vi "Dashboard Main.vi"() -> ()   [LabVIEW 2015]
uses:
  <vilib>/Utility/miscctls.llb/LVRowAndColumnTypeDef.ctl
  <vilib>/event_ctls.llb/eventvkey.ctl
  <vilib>/Rock Robotics/WPI/Dashboard/WPI_DashboardLogging Global.vi
  <vilib>/Rock Robotics/Network Tables/NT Read Numeric Array.vi
  <vilib>/Rock Robotics/Network Tables/SD Write Number.vi
  <vilib>/Rock Robotics/Network Tables/SD Write Boolean.vi
  <vilib>/Rock Robotics/Network Tables/NT Write Boolean.vi
  <vilib>/Utility/config.llb/Write Key (String).vi
  <vilib>/Utility/config.llb/Write Key (I32).vi
  <vilib>/Utility/config.llb/NI_LVConfig.lvlib
panel:
  in  "Vision 2":u16(ring)=3 items=["IP Camera"=3]
  out "Camera Image 2":T1(plugin-control)
  in  "TCP":refnum<k5>
  in  "Rec Mode":enum32{"Stop", "Record", "Playback"}(radio)
  in  "Vision":u16(ring)=1 items=["USB Cam"=1]
  out "Camera IP":string
  out "Image Message":string="Timeout in Camera Communications"
  in  "Dashboard Tab":T2(tab)
  out "X-Accelerometer":dbl
  in  "Select Auto":string(combo)
  out "NT Connection":bool
  in  "Camera Settings":T3={"Frame Rate"=30, "Compression"=30, "Size"=1} {"Frame Rate" scale=1.0..30.0; "Size" items=["640x480", "320x240", "160x120"]}
  out "MotorChart R":cluster{"Numeric":dbl, "Numeric":dbl}(graph)
  out "MotorChart L":T4(graph)
  out "MotorSliders R":cluster{"MotorSlide1":dbl, "MotorSlide2":dbl} {"MotorSlide2" scale=-1.0..1.0 scale format="%#_2e"; "MotorSlide1" scale=-1.0..1.0 scale format="%#_2e"}
  out "MotorSliders L":T5 {"MotorSlide4 2" scale=0.0..14.0 scale format="%#_2e"; "MotorSlide2" scale=-1.0..1.0 scale format="%#_2e"; "MotorSlide1" scale=-1.0..1.0 scale format="%#_2e"}
  out "JS1 Z":dbl(slide) scale=-1.0..1.0 scale format="%#_2e"
  out "JS1 Graph":cluster{"X":dbl, "Y":dbl}[](graph)
  out "JS1 Buttons":T6
  out "JS2 Z":dbl(slide) scale=-1.0..1.0 scale format="%#_2e"
  out "JS2 Graph":cluster{"X":dbl, "Y":dbl}[](graph)
  out "JS2 Buttons":T6
  out "Mode":T7(ring)=enum."Auto Disabled"
  in  "DB Camera Config":bool
  out "fps":dbl format="%#.1g"
  out "Mbps":dbl format="%#.1g"
  out "Mbps LED":bool
  out "Camera IP 2":string
  in  "Autonomous Select":T8(ring)
  in  "Speed Control":bool
  in  "Top Speed":dbl min=-1.0 max=1.0 step=0.01
  in  "Back Speed":dbl min=-1.0 max=1.0 step=0.01
  out "Gyro":dbl(knob) scale=0.0..360.0
  in  "Intake Speed":dbl min=-1.0 max=1.0 step=0.01
  in  "Gyro Reset":bool
  out "Z-Accelerometer":dbl
  out "Y-Accelerometer":dbl
  in  "DB/String 9":string
  in  "DB/String 8":string
  in  "DB/String 7":string
  in  "DB/String 6":string
  in  "DB/String 5":string
  in  "DB/String 4":string
  in  "DB/String 3":string
  in  "DB/String 2":string
  in  "DB/String 1":string
  in  "DB/String 0":string
  in  "DB/Slider 0":dbl(slide) scale=0.0..5.0
  in  "DB/Slider 1":dbl(slide) scale=0.0..5.0
  in  "DB/Slider 2":dbl(slide) scale=0.0..5.0
  in  "DB/Slider 3":dbl(slide) scale=0.0..5.0
  out "DB/LED 3":bool
  out "DB/LED 2":bool
  out "DB/LED 1":bool
  out "DB/LED 0":bool
  in  "DB/Button 3":bool
  in  "DB/Button 2":bool
  in  "DB/Button 1":bool
  in  "DB/Button 0":bool caption="New Name"
  out "Mbps 2":dbl format="%#.1g"
  in  "Camera Settings 2":T3={"Frame Rate"=30, "Compression"=30, "Size"=1} {"Frame Rate" scale=1.0..30.0; "Size" items=["640x480", "320x240", "160x120"]}
  out "fps 2":dbl format="%#.1g"
  in  "Rec Mode 2":enum32{"Stop", "Record", "Playback"}(radio)
  in  "Test Slider":dbl(slide) scale=0.0..100.0 scale format="%#_3g"
  in  "On/Off":bool caption="Solenoid"
  in  "Test Name":u16(ring) items=["Select the test to run..."]
  in  "Test Tree":string(tree)
  in  "Motor":cluster{"Value":dbl, "Enable":bool} {"Value" scale=-1.0..1.0 scale format="%#_3g"}
  out "Progress":T9 {"Test Progress" scale=0.0..100.0}
  in  "Rev/Fwd":cluster{"Forward":bool, "Reverse":bool}
  in  "Test Ring":u16(ring) items=["Monochrome", "Color"]
  out "Cmd Status":string
  in  "Execute Command":bool
  in  "Command Params":string[][](table)
  in  "Command Selection":i32(listbox)
  in  "CheckList":i32(listbox)
  out "Tree":string(tree)
  out "Camera Image":T1(plugin-control)
  out "Background":bool
  # "Left"
  # "Front"
  # "Right"
  # "Battery"
  # "This tab is a great place for autonomous settings and robot-specific values.\nPlace controls and indicators inside this tab and match name to\nDashboard Variables on robot. You can also delete this comment."
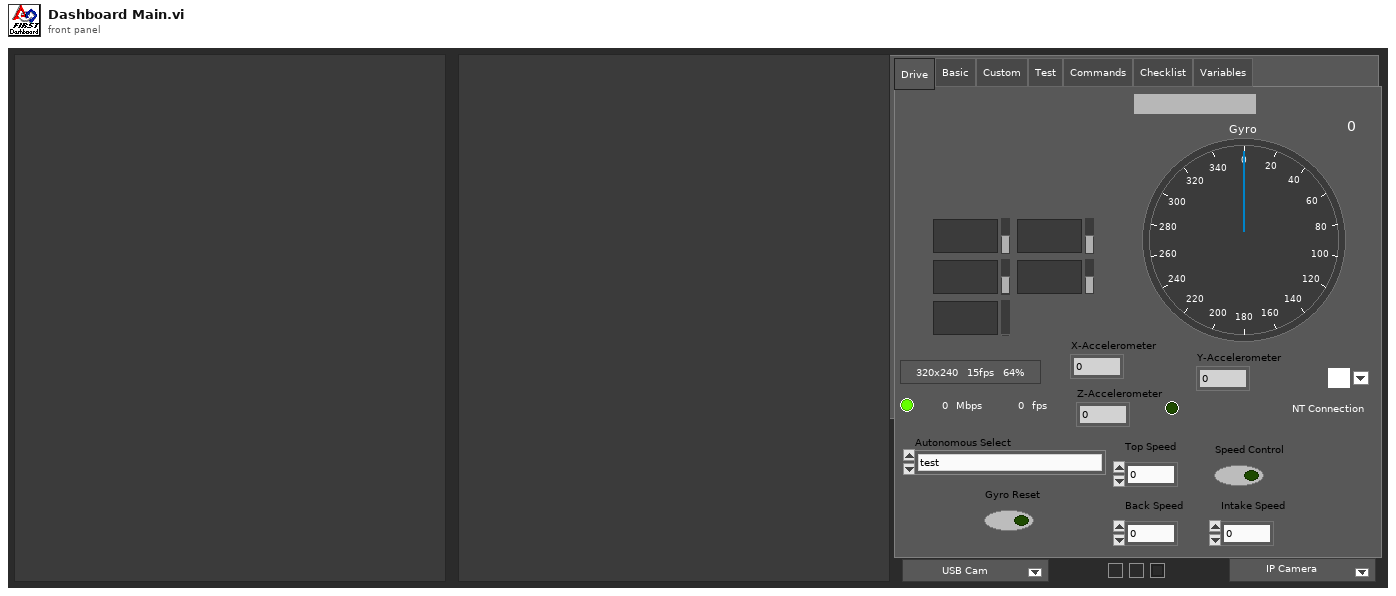
[diagram p1: front panel]
types:
  T1 = typedef "IMAQ Image.ctl" = refnum<image>
  T2 = enum32{"Drive", "Basic", "Custom", "Test", "Commands", "Checklist", "Variables"}
  T3 = cluster{"Frame Rate":i32, "Compression":i32, "Size":u16}
  T4 = cluster{"Numeric":dbl, "Numeric":dbl, "Battery V":dbl}
  T5 = cluster{"MotorSlide1":dbl, "MotorSlide2":dbl, "MotorSlide4 2":dbl}
  T6 = cluster{bool, bool, bool, bool, bool, bool, bool, bool, bool, bool, bool, bool}
  T7 = enum8{"Tele-Op Disabled", "Tele-Op Enabled", "Auto Disabled", "Auto Enabled", "Test Disabled", "Test Enabled", "Disconnected", "No Code", "E-Stop"}
  T8 = enum16{"test", "p value auto", "Ball Variable Shooter", "auto 3"}
  T9 = cluster{"Test Progress":u8, "Test Progress Text":string}
  T10 = typedef "Image Type" = u32
  T11 = cluster{"IDs":cluster{"RPC field ID":u16, "Unique ID":u16}, "String":string}
  T12 = enum32{"Drive", "Basic", "Custom", "Test", "Checklist", "Variables"}
  T13 = cluster{"Camera Image":refnum<vi>, "Dashboard Tab":refnum<vi>, "Background":refnum<vi>, "Vision":refnum<vi>, "Rec Mode":refnum<vi>, "Test Slider":refnum<vi>, "On/Off ":refnum<vi>, "Test Ring":refnum<vi>, "Rev/Fwd":refnum<vi>, "Test Name":refnum<vi>, "Motor":refnum<vi>, "Progress":refnum<vi>, "CheckList":refnum<vi>, "Tree":refnum<vi>, "Test Tree":refnum<vi>, "Command Params":refnum<vi>, "Command Selection":refnum<vi>, "Execute Command":refnum<vi>, "Cmd Status":refnum<vi>}
  T14 = typedef "NI_LVConfig.lvlib/Config Data RefNum.ctl" = refnum<k1>
  T15 = cluster{"Error Strings":string, "Disable Counts":cluster{u16, u16}, "Rail Faults":cluster{u16, u16, u16}, "Robot IP":string, "DB Mode":u8, "Event Info":cluster{"Name":string, "Type":u8, "Number":u16, "Replay":u8}, "Camera Addr":string}
  T16 = cluster{"Storage":cluster{"Disk Free":u64, "RAM Block":u32, "RAM free":u32}, "CPU Utilization":cluster{"CPU % ISR":sgl, "CPU % Time Crit":sgl, "CPU % Timed Str":sgl, "CPU % High":sgl, "CPU % Above":sgl, "CPU % Normal":sgl, "CPU % Low":sgl}, "CAN":cluster{"% Bus Utilization":sgl, "Bus Off Cnt":u32, "TX_FIFO Full Cnt":u32, "Receive Error Cnt":u8, "Transmit Error Cnt":u8}, "HID":cluster{"HID Outputs":u32, "Rumble Low":u16, "Rumble High":u16}[]}
  T17 = cluster{"Status bits":cluster{"Test Mode":bool, "Autonomous":bool, "Enabled":bool, "Code Start":bool, "Brownout":bool, "Reserved 2":bool, "Reserved 3":bool, "E-Stop":bool}, "Code Trace":cluster{"Disabled":bool, "TeleOp":bool, "Auto":bool, "Test":bool}, "Controller Type":enum16{"unknown", "cRIO", "roboRio"}, "Code?":enum16{"unknown", "noCode", "code"}, "Battery V":dbl}
  T18 = cluster{"Control Bits":cluster{"TestMode":bool, "Autonomous":bool, "Enabled":bool, "FMS Present":bool, bool, bool, bool, "E-Stop":bool}, "Team Station ":u8, "Countdown":sgl, "Joystick Values":cluster{"Axes":dbl[], "Buttons":bool[], "POVs":i16[]}[]}
  T19 = cluster{"Axes":dbl[], "Buttons":bool[], "POVs":i16[]}[]
  T20 = cluster{"Axes":dbl[], "Buttons":bool[], "POVs":i16[]}
  T21 = cluster{"Buttons[0]":bool, "Buttons[1]":bool, "Buttons[2]":bool, "Buttons[3]":bool, "Buttons[4]":bool, "Buttons[5]":bool, "Buttons[6]":bool, "Buttons[7]":bool, "Buttons[8]":bool, "Buttons[9]":bool, "Buttons[10]":bool, "Buttons[11]":bool}
  T22 = cluster{"Operation":enum16{"Update", "Clear"}, "Color Box":u32}[]
  T23 = typedef "eventvkey.ctl" = enum16{"ASCII", "Enter", "Return", "Shift", "Ctrl", "Alt", "Cmd", "Opt", "Caps", "NumLock", "Clear", "Break", "Up", "Down", "Left", "Right", "Insert", "Delete", "Home", "End", "PageUp", "PageDown", "Escape", "Help", "Pause", "ScrollLock", "F1", "F2", "F3", "F4", "F5", "F6", "F7", "F8", "F9", "F10", "F11", "F12", "F13", "F14", "F15", "F16", "F17", "F18", "F19", "F20", "F21", "F22", "F23", "F24", "Play", "VolumeUp", "VolumeDown", "Mute", "Two Byte Char"}
  T24 = cluster{"Image Size":bool, "Image Type":bool, "Pixel Value":bool, "ROI Information":bool, "Zoom Factor":bool}
  T25 = enum8{"Enabled", "Disabled", "Disabled and Grayed Out"}
  T26 = cluster{"Operation":enum16{"Update", "Clear"}, "Color Box":u32}
  T27 = typedef "LVRowAndColumnTypeDef.ctl" = cluster{"Row":i32, "Column":i32}
  T28 = cluster{"Shift":bool, "Ctrl":bool, "Alt":bool, "Cmd":bool, "Opt":bool}
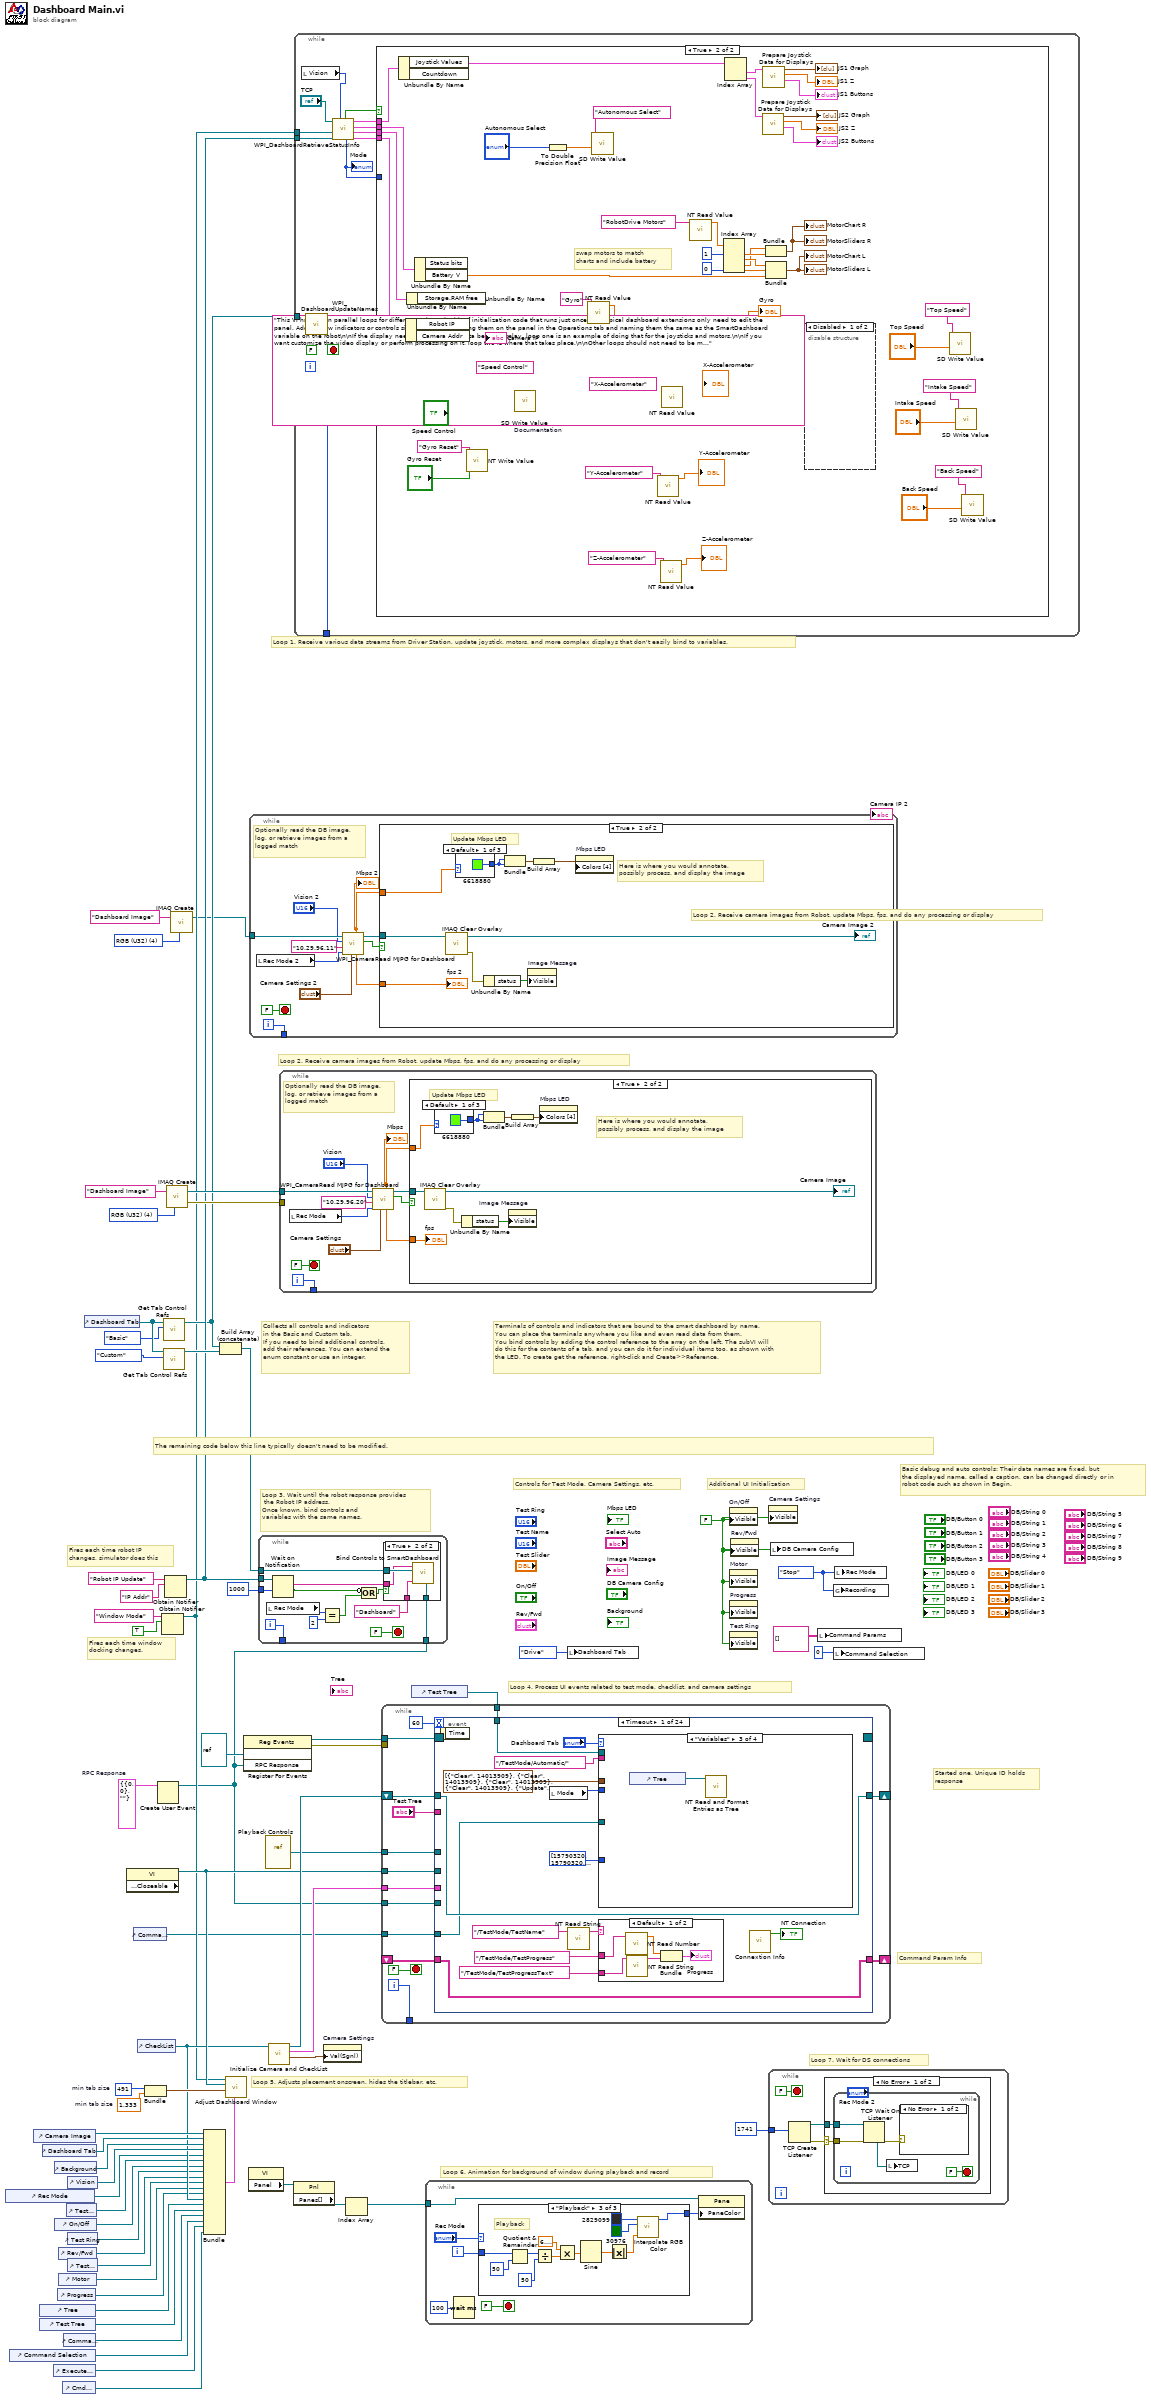
[diagram p0: block diagram]
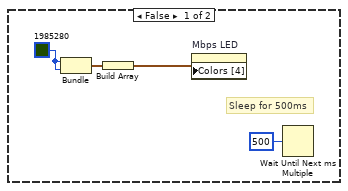
[diagram p2: hidden frame]
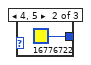
[diagram p3: hidden frame]
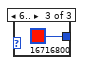
[diagram p4: hidden frame]
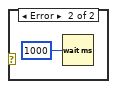
[diagram p5: hidden frame]
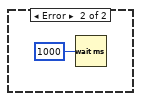
[diagram p6: hidden frame]
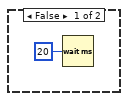
[diagram p7: hidden frame]
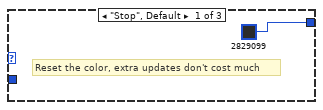
[diagram p9: hidden frame]
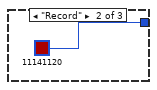
[diagram p10: hidden frame]
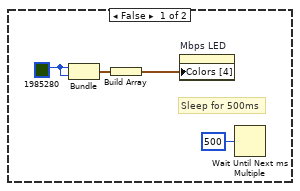
[diagram p12: hidden frame]
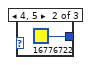
[diagram p13: hidden frame]
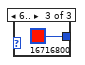
[diagram p14: hidden frame]
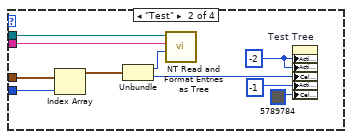
[diagram p16: hidden frame]
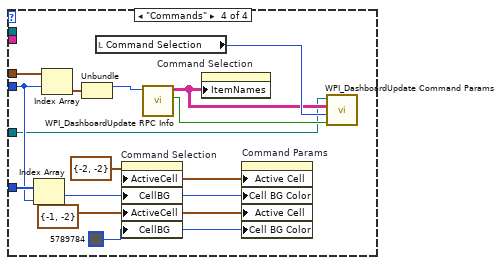
[diagram p17: hidden frame]
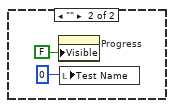
[diagram p18: hidden frame]
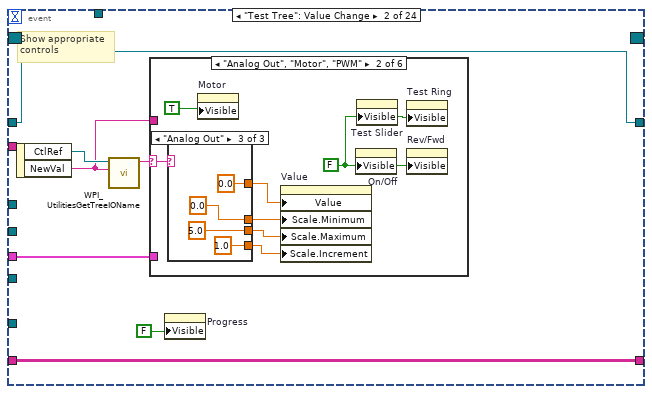
[diagram p19: hidden frame]
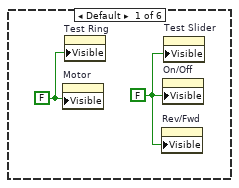
[diagram p20: hidden frame]
diagram:
  w2 = T10 4 items=["Grayscale (U8)", "Grayscale (I16)", "Grayscale (SGL)", "Complex (CSG)", "RGB (U32)", "HSL (U32)", "RGB (U64)"] ("Image Type")
  w10 = T11 {"IDs"={"RPC field ID"=0, "Unique ID"=0}, "String"=""}  # RPC Response
  w36 = 491  # min tab size
  w35 = 1.333  # min tab size
  w44 = enum32{"Stop", "Record", "Playback"}."Stop" ("Rec Mode")
  w18 = FALSE ("Visible")
  (unwired) "This VI has seven parallel loops for different tasks and a bit of initialization code that runs just once.\n\nTypical dashboard extensions only need to edit the panel. Adding new indicators or controls simply involves placing them on the panel in the Operations tab and naming them the same as the SmartDashboard variable on the robot\n\nIf the display needs to process the data before display, loop one is an example of doing that for the joysticks and motors.\n\nIf you want customize the video display or perform processing on it, loop two is where that takes place.\n\nOther loops should not need to be modified. They are pretty standard, and document the task they perform."  # Documentation
  w64 = T10 4 items=["Grayscale (U8)", "Grayscale (I16)", "Grayscale (SGL)", "Complex (CSG)", "RGB (U32)", "HSL (U32)", "RGB (U64)"] ("Image Type")
  # "Loop 2. Receive camera images from Robot, update Mbps, fps, and do any processing or display"
  # "Command Param Info"
  # "Started one, Unique ID holds\nresponse"
  # "Loop 7. Wait for DS connections"
  # "Basic debug and auto controls: Their data names are fixed, but\nthe displayed name, called a caption, can be changed directly or in\nrobot code such as shown in Begin."
  # "Controls for Test Mode, Camera Settings, etc."
  # "Additional UI Initialization"
  # "Loop 6. Animation for background of window during playback and record"
  # "Fires each time robot IP\nchanges, simulator does this"
  # "Fires each time window\ndocking changes."
  # "Collects all controls and indicators\nin the Basic and Custom tab.\nIf you need to bind additional controls,\nadd their references. You can extend the\nenum constant or use an integer."
  # "The remaining code below this line typically doesn't need to be modified."
  # "Loop 4. Process UI events related to test mode, checklist, and camera settings"
  # "Terminals of controls and indicators that are bound to the smart dashboard by name.\nYou can place the terminals anywhere you like and even read data from them.\nYou bind controls by adding the control reference to the array on the left. The subVI will\ndo this for the contents of a tab, and you can do it for individual items too, as shown with\nthe LED. To create get the reference, right-click and Create>>Reference."
  # "Loop 3. Wait until the robot response provides\n the Robot IP address.\nOnce known, bind controls and\nvariables with the same names."
  # "Loop 5. Adjusts placement onscreen, hides the titlebar, etc."
  # "Loop 1. Receive various data streams from Driver Station, update joystick, motors, and more complex displays that don't easily bind to variables."
  # "Loop 2. Receive camera images from Robot, update Mbps, fps, and do any processing or display"
  n1 = control-ref of="Rec Mode"() -> (w24:refnum<vi>)
  n2 = control-ref of="Command Selection"() -> (w9:refnum<vi>)
  n3 = control-ref of="Camera Image"() -> (w39:refnum<vi>)
  n4 = control-ref of="Tree"() -> (w28:refnum<vi>)
  n5 = control-ref of="Test Tree"() -> (w27:refnum<vi>)
  n6 = control-ref of="Dashboard Tab"() -> (w38:refnum<vi>)
  n7 = control-ref of="Execute Command"() -> (w11:refnum<vi>)
  n8 = control-ref of="Background"() -> (w33:refnum<vi>)
  n9 = control-ref of="On/Off"() -> (w22:refnum<vi>)
  n10 = control-ref of="Progress"() -> (w19:refnum<vi>)
  n11 = control-ref of="Rev/Fwd"() -> (w20:refnum<vi>)
  n12 = control-ref of="Motor"() -> (w25:refnum<vi>)
  n13 = control-ref of="Cmd Status"() -> (w5:refnum<vi>)
  n14 = control-ref of="Command Params"() -> (w12:refnum<vi>)
  n15 = control-ref of="Test Slider"() -> (w23:refnum<vi>)
  n16 = control-ref of="Vision"() -> (w37:refnum<vi>)
  n17 = control-ref of="Test Ring"() -> (w21:refnum<vi>)
  n18 = control-ref of="Test Name"() -> (w26:refnum<vi>)
  n19 = control-ref of="Dashboard Tab"() -> (w42:refnum<vi>)
  n20 = property class="VI" props=["Front Panel.Closeable"]() -> (reference out=w43:refnum<vi>)  [unwired: 2 in, 2 out]
  n21 = control-ref of="Command Params"() -> (w4:refnum<vi>)
  n22 = control-ref of="CheckList"() -> (w29:refnum<vi>)
  n23 = Bundle("min tab size"=w36, "min tab size"=w35) -> (w34:cluster{"min tab size":i32, "min tab size":dbl})  [unwired: 1 in]
  n24 = Create User Event(user event datatype=w10) -> (user event=w6:refnum<user-event>)  [unwired: 1 in, 1 out]
  n25 = Obtain Notifier(name (unnamed)="Window Mode", notification data type=TRUE) -> (notifier out=w15:refnum<notifier>)  [unwired: 2 in, 2 out]
  n26 = call <vilib>:"Get Tab Control Refs.vi"("Page Index"=T12."Basic" ("Dashboard Tab"), "TabControl in"=w42) -> ("ControlsOnPage"=w16:refnum<vi>[])  [unwired: 9 in]
  n27 = call <vilib>:"Get Tab Control Refs.vi"("Page Index"=T12."Custom" ("Dashboard Tab"), "TabControl in"=w42) -> ("ControlsOnPage"=w41:refnum<vi>[])  [unwired: 9 in]
  n28 = Obtain Notifier(name (unnamed)="Robot IP Update", notification data type="IP Addr" ("name (unnamed)")) -> (notifier out=w17:refnum<notifier>)  [unwired: 2 in, 2 out]
  n29 = call "IMAQ Create"("Image Name"="Dashboard Image", "Image Type"=w64) -> ("New Image"=w62:T1, "error out"=w61:errorcluster)  [unwired: 2 in, 1 out]
  n30 = call "IMAQ Create"("Image Name"="Dashboard Image", "Image Type"=w2) -> ("New Image"=w1:T1)  [unwired: 2 in, 2 out]
  n31 = Bundle("Camera Image"=w39, "Dashboard Tab"=w38, "Background"=w33, "Vision"=w37, "Rec Mode"=w24, "Test Slider"=w23, "On/Off"=w22, "Test Ring"=w21, "Rev/Fwd"=w20, "Test Name"=w26, "Motor"=w25, "Progress"=w19, "CheckList"=w29, "Tree"=w28, "Test Tree"=w27, "Command Params"=w12, "Command Selection"=w9, "Execute Command"=w11, "Cmd Status"=w5) -> (w30:T13)  [unwired: 1 in]
  n32 = Build Array (concatenate)(w16, w41) -> (w40:refnum<vi>[])
  n33 = call "Adjust Dashboard Window.vi"("Sizing Refnums"=w30, "Size Constraints"=w34, "VI"=w43, "WIn Mode"=w15) -> ()  [unwired: 8 in]
  n34 = register-events(refnum<vi> refnum, w6) -> (reference out=w48:refnum<event-registration>, error out=w47:errorcluster)  [unwired: 2 in]
  n35 = property class="VI"() -> ("Panel"=w51:refnum<vi>)  [unwired: 2 in, 2 out]
  n36 = while {
    tunnel: w1 -> [w73]
    tunnel: [w74] -> _
    i -> [w74]
    stop <- FALSE stop-if-true
    # "Optionally read the DB image,\nlog, or retrieve images from a\nlogged match"
    n37 = local read "Rec Mode 2"() -> (w68:enum32{"Stop", "Record", "Playback"})
    n38 = call <vilib>:"WPI_CameraRead MJPG for Dashboard.vi"("Camera Settings"="Camera Settings 2", "Rec Mode"=w68, "Camera IP"="10.29.96.11", "Camera Mode"="Vision 2", "Refnum in"=w73) -> ("Active"=w71:bool, "Refnum out"=w72:T1, "FPS"=w70:dbl, "Bandwidth (Mbps)"=w66:dbl)  [unwired: 3 in]
    "Mbps 2" <- w66
    n39 = case shown="True" w71 {
      tunnel: w72 -> [_ w85]
      tunnel: w66 -> [_ w84]
      tunnel: w70 -> [_ w82]
      frame False {
        w77 = u32 1985280 ("Color Box")
        # "Sleep for 500ms"
        n40 = Bundle("Color Box"=w77, "Color Box"=w77) -> (w78:cluster{"Color Box":u32, "Color Box":u32})  [unwired: 1 out]
        n41 = Build Array(w78) -> (w76:cluster{"Color Box":u32, "Color Box":u32}[])
        n42 = property on="Mbps LED" class="Bool (strict)"("Colors [4]"=w76) -> ()  [unwired: 2 in, 2 out]
        n43 = Wait Until Next ms Multiple(millisecond multiple=u32 500) -> ()  [unwired: 1 out]
      }
      frame True {
        # "Here is where you would annotate,\npossibly process, and display the image"
        # "Update Mbps LED"
        n44 = call "IMAQ Clear Overlay"("Image"=w85) -> ("error out"=w88:errorcluster, "Image Out"=→"Camera Image 2":T1)  [unwired: 2 in, 7 out]
        n45 = case shown="Default" w84 {
          tunnel: [u32 6618880 ("Color Box") u32 16776722 ("Color Box") u32 16716800 ("Color Box")] -> w86
          frame Default {
          }
          frame 4, 5 {
          }
          frame 6.. {
          }
        }
        n46 = Unbundle By Name(w88) -> ("status"=w80:bool)
        n47 = Bundle("Color Box"=w86, "Color Box"=w86) -> (w87:cluster{"Color Box":u32, "Color Box":u32})  [unwired: 1 out]
        n48 = property on="Image Message" class="Str"("Visible"=w80) -> ()  [unwired: 2 in, 2 out]
        n49 = Build Array(w87) -> (w81:cluster{"Color Box":u32, "Color Box":u32}[])
        n50 = property on="Mbps LED" class="Bool (strict)"("Colors [4]"=w81) -> ()  [unwired: 2 in, 2 out]
        "fps 2" <- w82
      }
    }
  }
  n51 = while {
    tunnel: w40 -> [w104]
    tunnel: w17 -> [w102]
    tunnel: [w100] -> _
    tunnel: u32 1000 ("milliseconds to wait") -> [w99]
    tunnel: w6 -> [w92]
    i -> [w100]
    stop <- FALSE stop-if-true
    n52 = local read "Rec Mode"() -> (w95:enum32{"Stop", "Record", "Playback"})
    n53 = Wait on Notification(notifier=w102, timeout in ms (-1)=w99) -> (notification=w101:string, timed out?=w97:bool)  [unwired: 2 in, 2 out]
    n54 = Equal?(x=w95, y=u16 2 ("Rec Mode")) -> (x = y?=w96:bool)
    n55 = Compound Arithmetic op=OR(invert w97, w96) -> (w98:bool)
    n56 = case shown="True" w98 {
      tunnel: w104 -> [_ w108]
      tunnel: w101 -> [_ w107]
      tunnel: "Dashboard" -> [_ w106]
      tunnel: w92 -> [_ w105]
      frame False {
      }
      frame True {
        n57 = call <vilib>:"Bind Controls to SmartDashboard.vi"("RPC ref"=w105, "Client Name"=w106, "Bound Control Refs"=w108, "Server IP Address"=w107) -> ()  [unwired: 8 in]
      }
    }
  }
  n58 = vi-ref "Playback Controls.vi"() -> (w49:refnum<vi>)
  n59 = call "Initialize Camera and CheckList.vi"("ListBox in"=w29) -> ("Cluster"=w55:cluster{"value":i32, "value":i32, "index":i32}, "Array"=w56:cluster{string[]}[], "File Refnum"=w54:T14)  [unwired: 8 in]
  n60 = while {
    tunnel: w62 -> [w117]
    tunnel: w61 -> [_]
    tunnel: [w118] -> _
    i -> [w118]
    stop <- FALSE stop-if-true
    # "Optionally read the DB image,\nlog, or retrieve images from a\nlogged match"
    n61 = local read "Rec Mode"() -> (w112:enum32{"Stop", "Record", "Playback"})
    n62 = call <vilib>:"WPI_CameraRead MJPG for Dashboard.vi"("Camera Settings"="Camera Settings", "Rec Mode"=w112, "Camera IP"="10.29.96.20", "Camera Mode"="Vision", "Refnum in"=w117) -> ("Active"=w115:bool, "Refnum out"=w116:T1, "FPS"=w114:dbl, "Bandwidth (Mbps)"=w110:dbl)  [unwired: 3 in]
    "Mbps" <- w110
    n63 = case shown="True" w115 {
      tunnel: w116 -> [_ w127]
      tunnel: w110 -> [_ w126]
      tunnel: w114 -> [_ w124]
      frame False {
        w120 = u32 1985280 ("Color Box")
        # "Sleep for 500ms"
        n64 = Bundle("Color Box"=w120, "Color Box"=w120) -> (w122:cluster{"Color Box":u32, "Color Box":u32})  [unwired: 1 out]
        n65 = Build Array(w122) -> (w121:cluster{"Color Box":u32, "Color Box":u32}[])
        n66 = property on="Mbps LED" class="Bool (strict)"("Colors [4]"=w121) -> ()  [unwired: 2 in, 2 out]
        n67 = Wait Until Next ms Multiple(millisecond multiple=u32 500) -> ()  [unwired: 1 out]
      }
      frame True {
        # "Here is where you would annotate,\npossibly process, and display the image"
        # "Update Mbps LED"
        n68 = call "IMAQ Clear Overlay"("Image"=w127) -> ("error out"=w131:errorcluster, "Image Out"=→"Camera Image":T1)  [unwired: 2 in, 7 out]
        n69 = case shown="Default" w126 {
          tunnel: [u32 6618880 ("Color Box") u32 16776722 ("Color Box") u32 16716800 ("Color Box")] -> w128
          frame Default {
          }
          frame 4, 5 {
          }
          frame 6.. {
          }
        }
        n70 = Unbundle By Name(w131) -> ("status"=w132:bool)
        n71 = Bundle("Color Box"=w128, "Color Box"=w128) -> (w130:cluster{"Color Box":u32, "Color Box":u32})  [unwired: 1 out]
        n72 = property on="Image Message" class="Str"("Visible"=w132) -> ()  [unwired: 2 in, 2 out]
        n73 = Build Array(w130) -> (w129:cluster{"Color Box":u32, "Color Box":u32}[])
        n74 = property on="Mbps LED" class="Bool (strict)"("Colors [4]"=w129) -> ()  [unwired: 2 in, 2 out]
        "fps" <- w124
      }
    }
  }
  n75 = property class="Pnl"(reference=w51) -> ("Panes[]"=w52:refnum<vi>[])  [unwired: 1 in, 2 out]
  n76 = while {
    tunnel: [w147] -> _
    tunnel: w17 -> [w141]
    tunnel: w16 -> [w140]
    tunnel: w15 -> [w136]
    i -> [w147]
    stop <- FALSE stop-if-true
    n77 = local read "Vision"() -> (w138:u16)
    n78 = call <vilib>:"WPI_DashboardUpdateNames.vi"("Controls on Tab"=w140) -> ()  [unwired: 11 in]
    n79 = call <vilib>:"WPI_DashboardRetrieveStatusInfo.vi"("Vision"=w138, "Binding Refnum"=w141, "Window Mode Notifier"=w136, "TCP Cnx"="TCP") -> ("Power and Errors"=w142:T15, "Robot Metrics"=w145:T16, "Status Info"=w146:T17, "Control Info"=w143:T18, "Robot Mode"=w139:T7, "Process?"=w144:bool)  [unwired: 2 in]
    "Mode" <- w139
    n80 = case shown="True" w144 {
      tunnel: w146 -> [_ w195]
      tunnel: w145 -> [_ w194]
      tunnel: w143 -> [_ w193]
      tunnel: w142 -> [_ w192]
      tunnel: w139 -> [_ _]
      frame False {
        n81 = Wait (ms)(milliseconds to wait=u32 20) -> ()  [unwired: 1 out]
      }
      frame True {
        # "swap motors to match\ncharts and include battery"
        n82 = Unbundle By Name(w193) -> ("Joystick Values"=w182:T19)  [unwired: 1 out]
        n83 = Unbundle By Name(w192) -> ("Camera Addr"=→"Camera IP":string)  [unwired: 1 out]
        n84 = Unbundle By Name(w194) -> ()  [unwired: 1 out]
        n85 = Unbundle By Name(w195) -> ("Battery V"=w183:dbl)  [unwired: 1 out]
        n86 = call-poly <vilib>:"NT Write Value.vi"("Boolean"="Gyro Reset", "Name"="Gyro Reset") -> ()  [unwired: 9 in, 1 out]
        n87 = call-poly <vilib>:"SD Write Value.vi"("Boolean"="Speed Control", "Name"="Speed Control") -> ()  [unwired: 8 in, 2 out]
        n88 = To Double Precision Float(number="Autonomous Select") -> (double precision float=w168:dbl)
        n89 = call-poly <vilib>:"NT Read Value.vi"("Name"="Gyro") -> ("Numeric"=→"Gyro":dbl)  [unwired: 9 in, 1 out]
        n90 = call-poly <vilib>:"SD Write Value.vi"("Numeric"=w168, "Name"="Autonomous Select") -> ()  [unwired: 8 in, 2 out]
        n91 = call-poly <vilib>:"NT Read Value.vi"("Name"="Y-Accelerometer") -> ("Numeric"=→"Y-Accelerometer":dbl)  [unwired: 9 in, 1 out]
        n92 = call-poly <vilib>:"NT Read Value.vi"("Name"="Z-Accelerometer") -> ("Numeric"=→"Z-Accelerometer":dbl)  [unwired: 9 in, 1 out]
        n93 = call-poly <vilib>:"NT Read Value.vi"("Name"="X-Accelerometer") -> ("Numeric"=→"X-Accelerometer":dbl)  [unwired: 9 in, 1 out]
        n94 = call-poly <vilib>:"NT Read Value.vi"("Name"="RobotDrive Motors") -> ("Numeric Array"=w171:dbl[])  [unwired: 9 in, 1 out]
        n95 = Index Array(array=w171, index #1=1, index #4=0) -> (element #1=w187:dbl, element #2=w188:dbl, element #3=w186:dbl, element #4=w191:dbl)  [unwired: 2 in]
        n96 = Index Array(array=w182) -> (element #1=w181:T20, element #2=w176:T20)  [unwired: 2 in]
        n97 = call "Prepare Joystick Data for Displays.vi"("Joystick Values"=w176) -> ("Buttons"=→"JS2 Buttons":T21, "Z Axis"=→"JS2 Z":dbl, "Cartesian Data"=→"JS2 Graph":cluster{"X axis":dbl, "X axis":dbl}[])  [unwired: 8 in]
        n98 = call "Prepare Joystick Data for Displays.vi"("Joystick Values"=w181) -> ("Buttons"=→"JS1 Buttons":T21, "Z Axis"=→"JS1 Z":dbl, "Cartesian Data"=→"JS1 Graph":cluster{"X axis":dbl, "X axis":dbl}[])  [unwired: 8 in]
        n99 = Bundle("Numeric"=w186, "Numeric"=w187) -> (→"MotorChart R" →"MotorSliders R":cluster{"Numeric":dbl, "Numeric":dbl})  [unwired: 1 in]
        n100 = Bundle("Numeric"=w188, "Numeric"=w191, "Battery V"=w183) -> (→"MotorChart L" →"MotorSliders L":T4)  [unwired: 1 in]
        n101 = disable-structure shown="Disabled" {
          frame Disabled {
          }
          frame Enabled {
          }
        }
        n102 = call-poly <vilib>:"SD Write Value.vi"("Numeric"="Top Speed", "Name"="Top Speed") -> ()  [unwired: 8 in, 2 out]
        n103 = call-poly <vilib>:"SD Write Value.vi"("Numeric"="Intake Speed", "Name"="Intake Speed") -> ()  [unwired: 8 in, 2 out]
        n104 = call-poly <vilib>:"SD Write Value.vi"("Numeric"="Back Speed", "Name"="Back Speed") -> ()  [unwired: 8 in, 2 out]
      }
    }
  }
  n105 = property on="Camera Settings" class="Clust (strict)"("Val(Sgnl)"=w55) -> ()  [unwired: 2 in, 2 out]
  n106 = Index Array(array=w52) -> (element=w50:refnum<vi>)  [unwired: 1 in]
  n107 = control-ref of="Test Tree"() -> (w53:refnum<vi>)
  n108 = while {
    tunnel: w56 -> [w207]
    shift-right: [w206] -> _
    shift-left: w54 -> [w205]
    tunnel: [w204] -> _
    tunnel: w53 -> [w203]
    tunnel: w49 -> [w202]
    tunnel: w48 -> [w201]
    tunnel: w47 -> [_]
    tunnel: w43 -> [w200]
    tunnel: w6 -> [w199]
    tunnel: w4 -> [w198]
    shift-right: [w197] -> _
    shift-left: _ -> [w196]
    i -> [w204]
    stop <- FALSE stop-if-true
    n109 = event shown="[0] Timeout" {
      selector: w201 -> [_ _ _ _ _ _ _ _ _ _ _ _ _ _ _ _ _ _ _ _ _ _ _ _]
      dyn-events: [_ _ _ _ _ _ _ _ _ _ _ _ _ _ _ _ _ _ w516 _ _ _ _ _] -> _
      timeout: u32 60 ("milliseconds to wait") -> [_ _ _ _ _ _ _ _ _ _ _ _ _ _ _ _ _ _ _ _ _ _ _ _]
      tunnel: w203 -> [w220 _ _ _ _ _ _ _ _ _ _ _ _ _ _ _ _ _ _ _ _ _ _ _]
      tunnel: "Test Tree" -> [_ _ _ _ _ _ _ _ _ _ _ _ _ w479 w488 w491 w496 w505 _ _ _ _ _ _]
      tunnel: w207 -> [_ w258 _ _ _ _ _ _ _ _ _ w441 w472 _ _ _ _ _ _ _ _ _ _ _]
      tunnel: [w217 w257 w361 w367 w377 w381 w387 w399 w407 w413 w426 w440 w465 w478 w486 w490 w495 w504 w518 w534 w536 w544 w555 w560] -> w206
      tunnel: w205 -> [w217 w257 w361 w367 w377 w381 w387 w399 w407 w413 w426 w439 w465 w478 w486 w490 w495 w504 w518 w534 w536 w544 w555 w560]
      tunnel: w202 -> [_ _ _ _ _ _ _ _ _ _ _ _ _ _ _ _ _ _ w519 _ w539 _ _ _]
      tunnel: w200 -> [_ _ _ _ _ _ _ _ _ _ _ _ _ _ _ _ _ _ w514 _ _ _ _ _]
      tunnel: w199 -> [_ _ _ _ _ _ _ _ _ _ _ _ _ _ _ _ _ _ w510 _ _ _ _ _]
      tunnel: w198 -> [w212 _ _ _ _ _ w385 _ _ _ _ _ _ _ _ _ _ _ _ _ _ _ _ _]
      tunnel: [w211 w256 w360 w366 w376 w382 w383 w393 w404 w412 w425 w438 w464 w477 w485 w489 w494 w503 w509 w532 w535 w540 w548 w561] -> w197
      tunnel: w196 -> [w211 w256 w360 w366 w376 w382 w383 _ _ w412 w425 w438 w464 w477 w485 w489 w494 w503 w509 w532 w535 w540 w548 w561]
      event Timeout {
        n110 = event-data() -> ()  [unwired: 1 in, 1 out]
        n111 = local read "Mode"() -> (w214:T7)
        n112 = call <vilib>:"NT Read String.vi"("Name"="/TestMode/TestName") -> ("String"=w223:string)  [unwired: 9 in, 1 out]
        n113 = case shown="\"Variables\"" "Dashboard Tab" {
          tunnel: w220 -> [_ w234 _ _]
          tunnel: "/TestMode/Automatic/" ("Name Pattern") -> [_ w233 _ _]
          tunnel: T22 [{"Operation"=enum."Clear", "Color Box"=14013909}, {"Operation"=enum."Clear", "Color Box"=14013909}, {"Operation"=enum."Clear", "Color Box"=14013909}, {"Operation"=enum."Clear", "Color Box"=14013909}, {"Operation"=enum."Update", "Color Box"=14013909}, {"Operation"=enum."Update", "Color Box"=16777215}, {"Operation"=enum."Clear", "Color Box"=14013909}, {"Operation"=enum."Clear", "Color Box"=14013909}, {"Operation"=enum."Clear", "Color Box"=14013909}] -> [_ w226 _ w243]
          tunnel: w214 -> [_ w225 _ w242]
          tunnel: u32[] [15790320, 15790320, 15790320, 15790320, 16777215, 16777215, 15790320, 15790320, 15790320] -> [_ _ _ w248]
          tunnel: w212 -> [_ _ _ w236]
          frame "Custom", Default {
          }
          frame "Test" {
            w232 = -2 ("Active Item:Row Number")
            n114 = Index Array(array=w226, index=w225) -> (element=w227:T26)
            n115 = Unbundle(w227) -> ("Operation"=w228:enum16{"Update", "Clear"}, "Color Box"=w229:u32)
            n116 = call <vilib>:"NT Read and Format Entries as Tree.vi"("Operation"=w228, "Name Pattern"=w233, "Tree Refnum"=w234) -> ()  [unwired: 7 in, 2 out]
            n117 = property on="Test Tree" class="Tree (strict)"("Active Item Row Number"=w232, "ActiveColNum"=w232, "CellBG"=w229, "Active Item Row Number"=-1 ("Active Item:Row Number"), "CellBG"=u32 5789784 ("Color Box")) -> ()  [unwired: 2 in, 2 out]
          }
          frame "Variables" {
            n118 = control-ref of="Tree"() -> (w235:refnum<vi>)
            n119 = call <vilib>:"NT Read and Format Entries as Tree.vi"("Tree Refnum"=w235) -> ()  [unwired: 9 in, 2 out]
          }
          frame "Commands" {
            w244 = u32 5789784 ("Color Box")
            w245 = T27 {"Row"=-1, "Column"=-2} ("Active Cell:Active Cell")
            w247 = T27 {"Row"=-2, "Column"=-2} ("Active Cell:Active Cell")
            n120 = Index Array(array=w248, index=w242) -> (element=w246:u32)
            n121 = Index Array(array=w243, index=w242) -> (element=w241:T26)
            n122 = Unbundle(w241) -> ("Operation"=w240:enum16{"Update", "Clear"})  [unwired: 1 out]
            n123 = local read "Command Selection"() -> (w239:i32)
            n124 = property on="Command Selection" class="MCListbox (strict)"("ActiveCell"=w247, "CellBG"=w246, "ActiveCell"=w245, "CellBG"=w244) -> ()  [unwired: 2 in, 2 out]
            n125 = call <vilib>:"WPI_DashboardUpdate RPC Info.vi"("Operation"=w240) -> ("update"=w238:bool, "commands"=w237:string[][])  [unwired: 9 in]
            n126 = property on="Command Selection" class="MCListbox (strict)"("ItemNames"=w237) -> ()  [unwired: 2 in, 2 out]
            n127 = property on="Command Params" class="Tbl (strict)"("Active Cell"=w247, "Cell BG Color"=w246, "Active Cell"=w245, "Cell BG Color"=w244) -> ()  [unwired: 2 in, 2 out]
            n128 = call <vilib>:"WPI_DashboardUpdate Command Params.vi"("Update"=w238, "NewVal"=w239, "Commands"=w237, "Param Tbl"=w236) -> ()  [unwired: 7 in, 1 out]
          }
        }
        n129 = case shown="Default" w223 {
          tunnel: "/TestMode/TestProgress" ("Name") -> [w250 _]
          tunnel: "/TestMode/TestProgressText" ("Name") -> [w249 _]
          frame Default {
            n130 = call <vilib>:"NT Read Number.vi"("Name"=w250) -> ("Numeric"=w251:dbl)  [unwired: 9 in, 1 out]
            n131 = call <vilib>:"NT Read String.vi"("Name"=w249) -> ("String"=w252:string)  [unwired: 9 in, 1 out]
            n132 = Bundle("Numeric"=w251, "String"=w252) -> (→"Progress":cluster{"Numeric":dbl, "String":string})  [unwired: 1 in]
          }
          frame "" {
            n133 = property on="Progress" class="Clust (strict)"("Visible"=FALSE) -> ()  [unwired: 2 in, 2 out]
            n134 = local write "Test Name"(u16 0) -> ()
          }
        }
        n135 = call <vilib>:"Connextion Info.vi"() -> ("Connected"=→"NT Connection":bool)  [unwired: 10 in, 1 out]
      }
      event "Test Tree": Value Change {
        # "Show appropriate\ncontrols"
        n136 = event-data() -> ("CtlRef"=w261:refnum<vi>, "NewVal"=w259:string)  [unwired: 1 in]
        n137 = call <vilib>:"WPI_UtilitiesGetTreeIOName.vi"("NewVal"=w259, "TreeControl in"=w261) -> ("I/O Name"=w262:string)  [unwired: 9 in]
        n138 = case shown="\"Analog Out\", \"Motor\", \"PWM\"" w262 {
          selector: w262 -> [_ w269 _ w291 w300 _]
          tunnel: w259 -> [_ _ w288 w290 _ w307]
          tunnel: w258 -> [_ _ _ _ _ w306]
          frame Default {
            w264 = FALSE ("Visible")
            w263 = FALSE ("Visible")
            n139 = property on="Motor" class="Clust (strict)"("Visible"=w263) -> ()  [unwired: 2 in, 2 out]
            n140 = property on="Test Ring" class="Ring (strict)"("Visible"=w263) -> ()  [unwired: 2 in, 2 out]
            n141 = property on="Rev/Fwd" class="Clust (strict)"("Visible"=w264) -> ()  [unwired: 2 in, 2 out]
            n142 = property on="On/Off" class="Bool (strict)"("Visible"=w264) -> ()  [unwired: 2 in, 2 out]
            n143 = property on="Test Slider" class="Slide (strict)"("Visible"=w264) -> ()  [unwired: 2 in, 2 out]
          }
          frame "Analog Out", "Motor", "PWM" {
            w270 = FALSE ("Visible")
            n144 = case shown="\"Analog Out\"" w269 {
              tunnel: [1.0 ("Value") -1.0 ("Value") 0.0 ("Value")] -> w268
              tunnel: [255.0 ("Value") 1.0 ("Value") 5.0 ("Value")] -> w267
              tunnel: [128.0 ("Value") 0.0 ("Value") 0.0 ("Value")] -> w266
              tunnel: [64.0 ("Value") 0.5 ("Value") 1.0 ("Value")] -> w265
              frame "PWM" {
              }
              frame "Motor", Default {
              }
              frame "Analog Out" {
              }
            }
            n145 = property on="Motor" class="Clust (strict)"("Visible"=TRUE) -> ()  [unwired: 2 in, 2 out]
            n146 = property on="Value" class="Slide (strict)"("Value"=w266, "Scale.Minimum"=w268, "Scale.Maximum"=w267, "Scale.Increment"=w265) -> ()  [unwired: 2 in, 2 out]
            n147 = property on="On/Off" class="Bool (strict)"("Visible"=w270) -> ()  [unwired: 2 in, 2 out]
            n148 = property on="Test Slider" class="Slide (strict)"("Visible"=w270) -> ()  [unwired: 2 in, 2 out]
            n149 = property on="Test Ring" class="Ring (strict)"("Visible"=w270) -> ()  [unwired: 2 in, 2 out]
            n150 = property on="Rev/Fwd" class="Clust (strict)"("Visible"=w270) -> ()  [unwired: 2 in, 2 out]
          }
          frame "Servo" {
            w286 = FALSE ("Visible")
            n151 = call <vilib>:"NT Read Number.vi"("Name"=w288) -> ("Numeric"=w287:dbl)  [unwired: 9 in, 1 out]
            n152 = property on="Test Slider" class="Slide (strict)"("Visible"=TRUE, "Scale.Maximum"=170.0 ("Scale.Range:Maximum")) -> ()  [unwired: 2 in, 2 out]
            n153 = local write "Test Slider"(w287) -> ()
            n154 = property on="Motor" class="Clust (strict)"("Visible"=w286) -> ()  [unwired: 2 in, 2 out]
            n155 = property on="Rev/Fwd" class="Clust (strict)"("Visible"=w286) -> ()  [unwired: 2 in, 2 out]
            n156 = property on="On/Off" class="Bool (strict)"("Visible"=w286) -> ()  [unwired: 2 in, 2 out]
            n157 = property on="Test Ring" class="Ring (strict)"("Visible"=w286) -> ()  [unwired: 2 in, 2 out]
          }
          frame "Relay", "Solenoid" {
            w289 = FALSE ("Visible")
            n158 = property on="Motor" class="Clust (strict)"("Visible"=w289) -> ()  [unwired: 2 in, 2 out]
            n159 = property on="Test Slider" class="Slide (strict)"("Visible"=w289) -> ()  [unwired: 2 in, 2 out]
            n160 = Search and Replace String(input string=w290, search string="/Value  **", replace string="/Direction") -> (result string=w296:string)  [unwired: 5 in, 3 out]
            n161 = property on="Test Ring" class="Ring (strict)"("Visible"=w289) -> ()  [unwired: 2 in, 2 out]
            n162 = call <vilib>:"NT Read String.vi"("Name"=w296) -> ("String"=w294:string)  [unwired: 9 in, 1 out]
            n163 = Equal?(x="Both directions", y=w294) -> (x = y?=w292:bool)
            n164 = Not(x=w292) -> (.not. x?=w293:bool)
            n165 = property on="Rev/Fwd" class="Clust (strict)"("Visible"=w292) -> ()  [unwired: 2 in, 2 out]
            n166 = property on="On/Off" class="Bool (strict)"("Visible"=w293, "Caption.Text"=w291) -> ()  [unwired: 2 in, 2 out]
          }
          frame "Compressor", "Digital Out" {
            w299 = FALSE ("Visible")
            # "Get direction and finish"
            n167 = property on="Motor" class="Clust (strict)"("Visible"=w299) -> ()  [unwired: 2 in, 2 out]
            n168 = property on="Test Slider" class="Slide (strict)"("Visible"=w299) -> ()  [unwired: 2 in, 2 out]
            n169 = property on="Test Ring" class="Ring (strict)"("Visible"=w299) -> ()  [unwired: 2 in, 2 out]
            n170 = property on="On/Off" class="Bool (strict)"("Visible"=TRUE, "Caption.Text"=w300) -> ()  [unwired: 2 in, 2 out]
            n171 = property on="Rev/Fwd" class="Clust (strict)"("Visible"=FALSE) -> ()  [unwired: 2 in, 2 out]
          }
          frame "Camera" {
            n172 = call <vilib>:"Get Last Path Segment.vi"("String in"=w307) -> ("String out"=w308:string)  [unwired: 10 in]
            n173 = property on="On/Off" class="Bool (strict)"("Visible"=FALSE) -> ()  [unwired: 2 in, 2 out]
            n174 = property on="Motor" class="Clust (strict)"("Visible"=FALSE) -> ()  [unwired: 2 in, 2 out]
            n175 = property on="Rev/Fwd" class="Clust (strict)"("Visible"=FALSE) -> ()  [unwired: 2 in, 2 out]
            n176 = case shown="\"White Balance  **\"" w308 {
              tunnel: w307 -> [w314 w323 w332 w341 w350 _ w356]
              tunnel: w306 -> [w312 w320 w329 w338 w347 _ _]
              frame "Size  **" {
                n177 = Index Array(array=w312) -> (element=w311:cluster{string[]})  [unwired: 1 in]
                n178 = call <vilib>:"NT Read String.vi"("Name"=w314) -> ("String"=w313:string)  [unwired: 9 in, 1 out]
                n179 = Unbundle(w311) -> (w309:string[])
                n180 = Match First String(2:w309, 3:w313) -> (0:w310:i32)  [unwired: 1 out]
                n181 = property on="Test Ring" class="Ring (strict)"("Value"=w310, "Strings []"=w309) -> ()  [unwired: 2 in, 2 out]
                n182 = property on="Test Ring" class="Ring (strict)"("Visible"=TRUE) -> ()  [unwired: 2 in, 2 out]
                n183 = property on="Test Slider" class="Slide (strict)"("Visible"=FALSE) -> ()  [unwired: 2 in, 2 out]
              }
              frame "White Balance  **" {
                n184 = Index Array(array=w320, index=1) -> (element=w321:cluster{string[]})
                n185 = call <vilib>:"NT Read String.vi"("Name"=w323) -> ("String"=w322:string)  [unwired: 9 in, 1 out]
                n186 = Unbundle(w321) -> (w318:string[])
                n187 = Match First String(2:w318, 3:w322) -> (0:w317:i32)  [unwired: 1 out]
                n188 = property on="Test Ring" class="Ring (strict)"("Value"=w317, "Strings []"=w318) -> ()  [unwired: 2 in, 2 out]
                n189 = property on="Test Ring" class="Ring (strict)"("Visible"=TRUE) -> ()  [unwired: 2 in, 2 out]
                n190 = property on="Test Slider" class="Slide (strict)"("Visible"=FALSE) -> ()  [unwired: 2 in, 2 out]
              }
              frame "Exposure  **" {
                n191 = Index Array(array=w329, index=2) -> (element=w330:cluster{string[]})
                n192 = call <vilib>:"NT Read String.vi"("Name"=w332) -> ("String"=w331:string)  [unwired: 9 in, 1 out]
                n193 = Unbundle(w330) -> (w326:string[])
                n194 = Match First String(2:w326, 3:w331) -> (0:w327:i32)  [unwired: 1 out]
                n195 = property on="Test Ring" class="Ring (strict)"("Value"=w327, "Strings []"=w326) -> ()  [unwired: 2 in, 2 out]
                n196 = property on="Test Ring" class="Ring (strict)"("Visible"=TRUE) -> ()  [unwired: 2 in, 2 out]
                n197 = property on="Test Slider" class="Slide (strict)"("Visible"=FALSE) -> ()  [unwired: 2 in, 2 out]
              }
              frame "Exposure Priority  **" {
                n198 = Index Array(array=w338, index=3) -> (element=w339:cluster{string[]})
                n199 = call <vilib>:"NT Read String.vi"("Name"=w341) -> ("String"=w340:string)  [unwired: 9 in, 1 out]
                n200 = Unbundle(w339) -> (w335:string[])
                n201 = Match First String(2:w335, 3:w340) -> (0:w336:i32)  [unwired: 1 out]
                n202 = property on="Test Ring" class="Ring (strict)"("Value"=w336, "Strings []"=w335) -> ()  [unwired: 2 in, 2 out]
                n203 = property on="Test Ring" class="Ring (strict)"("Visible"=TRUE) -> ()  [unwired: 2 in, 2 out]
                n204 = property on="Test Slider" class="Slide (strict)"("Visible"=FALSE) -> ()  [unwired: 2 in, 2 out]
              }
              frame "Color Enable  **" {
                n205 = Index Array(array=w347, index=4) -> (element=w348:cluster{string[]})
                n206 = call <vilib>:"NT Read String.vi"("Name"=w350) -> ("String"=w349:string)  [unwired: 9 in, 1 out]
                n207 = Unbundle(w348) -> (w344:string[])
                n208 = Match First String(2:w344, 3:w349) -> (0:w345:i32)  [unwired: 1 out]
                n209 = property on="Test Ring" class="Ring (strict)"("Value"=w345, "Strings []"=w344) -> ()  [unwired: 2 in, 2 out]
                n210 = property on="Test Ring" class="Ring (strict)"("Visible"=TRUE) -> ()  [unwired: 2 in, 2 out]
                n211 = property on="Test Slider" class="Slide (strict)"("Visible"=FALSE) -> ()  [unwired: 2 in, 2 out]
              }
              frame Default {
                n212 = property on="Test Ring" class="Ring (strict)"("Visible"=FALSE) -> ()  [unwired: 2 in, 2 out]
                n213 = property on="Test Slider" class="Slide (strict)"("Visible"=FALSE) -> ()  [unwired: 2 in, 2 out]
              }
              frame "Brightness  **", "Color Level  **", "Compression  **", "FPS  **", "Sharpness  **" {
                n214 = call <vilib>:"NT Read Number.vi"("Name"=w356) -> ("Numeric"=w355:dbl)  [unwired: 9 in, 1 out]
                n215 = local write "Test Slider"(w355) -> ()
                n216 = property on="Test Slider" class="Slide (strict)"("Visible"=TRUE, "Scale.Maximum"=100.0 ("Scale.Range:Maximum")) -> ()  [unwired: 2 in, 2 out]
                n217 = property on="Test Ring" class="Ring (strict)"("Visible"=FALSE) -> ()  [unwired: 2 in, 2 out]
              }
            }
          }
        }
        n218 = property on="Progress" class="Clust (strict)"("Visible"=FALSE) -> ()  [unwired: 2 in, 2 out]
      }
      event "Test Name": Mouse Enter {
        # "Populate the ring with the list of tests"
        n219 = event-data() -> ()  [unwired: 1 in, 1 out]
        n220 = call <vilib>:"NT Read String Array.vi"("Name"="/TestMode/TestList") -> ("String Array"=w365:string[])  [unwired: 9 in, 1 out]
        n221 = Build Array (concatenate)("Select the test to run...", w365) -> (w364:string[])
        n222 = property on="Test Name" class="Ring (strict)"("Strings []"=w364) -> ()  [unwired: 2 in, 2 out]
      }
      event "Test Name": Value Change {
        w368 = FALSE ("Visible")
        # "Tell the robot the test name to run"
        n223 = event-data() -> ("NewVal"=w372:u16)  [unwired: 1 in]
        n224 = property on="Test Name" class="Ring (strict)"() -> ("Strings []"=w373:string[])  [unwired: 2 in, 2 out]
        n225 = local write "Progress"(T9 {"Test Progress"=0, "Test Progress Text"=""} ("Progress")) -> ()
        n226 = Index Array(array=w373, index=w372) -> (element=w371:string)
        n227 = call <vilib>:"NT Write String.vi"("String"=w371, "Name"="/TestMode/TestName") -> ()  [unwired: 9 in, 1 out]
        n228 = property on="Progress" class="Clust (strict)"("Visible"=TRUE) -> ()  [unwired: 2 in, 2 out]
        n229 = property on="Motor" class="Clust (strict)"("Visible"=w368) -> ()  [unwired: 2 in, 2 out]
        n230 = property on="Test Slider" class="Slide (strict)"("Visible"=w368) -> ()  [unwired: 2 in, 2 out]
        n231 = property on="On/Off" class="Bool (strict)"("Visible"=w368) -> ()  [unwired: 2 in, 2 out]
        n232 = property on="Rev/Fwd" class="Clust (strict)"("Visible"=w368) -> ()  [unwired: 2 in, 2 out]
        n233 = property on="Test Ring" class="Ring (strict)"("Visible"=w368) -> ()  [unwired: 2 in, 2 out]
      }
      event "Select Auto": Mouse Enter {
        # "Populate the combo box with the list of autonomous options"
        n234 = event-data() -> ()  [unwired: 1 in, 1 out]
        n235 = call <vilib>:"NT Read String Array.vi"("Name"="Auto List") -> ("String Array"=w375:string[])  [unwired: 9 in, 1 out]
        n236 = property on="Select Auto" class="CmbBox"("Strings[]"=w375) -> ()  [unwired: 2 in, 2 out]
      }
      event "Select Auto": Value Change {
        # "User modified the Auto Selection. Write to NT variable so robot knows."
        n237 = event-data() -> ("NewVal"=w379:string)  [unwired: 1 in]
        n238 = call <vilib>:"NT Write String.vi"("String"=w379, "Name"="Auto Selector") -> ()  [unwired: 9 in, 1 out]
      }
      event "Command Selection": Value Change {
        # "Get the params and show in table"
        n239 = event-data() -> ("NewVal"=w386:i32)  [unwired: 1 in]
        n240 = property on="Command Selection" class="MCListbox (strict)"() -> ("ItemNames"=w384:string[][])  [unwired: 2 in, 2 out]
        n241 = call <vilib>:"WPI_DashboardUpdate Command Params.vi"("NewVal"=w386, "Commands"=w384, "Param Tbl"=w385) -> ()  [unwired: 8 in, 1 out]
      }
      event "Execute Command": Value Change {
        # "Started one, Unique ID holds\nresponse"
        n242 = event-data() -> ()  [unwired: 1 in, 1 out]
        n243 = property on="Command Selection" class="MCListbox (strict)"() -> ("ItemNames"=w398:string[][])  [unwired: 2 in, 2 out]
        n244 = Index Array(array=w398, index (row)="Command Selection", index (col)=0) -> (element=w396:string)
        n245 = call <vilib>:"Invoke Commands.vi"("Command Params"="Command Params", "Function Name"=w396) -> ("Params"=w392:u8, "Started"=w391:bool)  [unwired: 7 in, 1 out]
        n246 = Array Subset(array="Command Params", length (row)=w392) -> (w393:string[][])  [unwired: 3 in]
        n247 = Select(t="Executing" ("Cmd Status"), s=w391, f="" ("Cmd Status")) -> (s? t:f=→"Cmd Status":string)
      }
      event "Command Selection": Double Click {
        n248 = event-data() -> ("Row"=w408:i32)  [unwired: 1 in]
        n249 = property on="Command Selection" class="MCListbox (strict)"() -> ("ItemNames"=w411:string[][])  [unwired: 2 in, 2 out]
        n250 = local read "Command Params"() -> (w406:string[][])
        n251 = Index Array(array=w411, index (row)=w408, index (col)=0) -> (element=w409:string)
        n252 = call <vilib>:"Invoke Commands.vi"("Command Params"=w406, "Function Name"=w409) -> ("Params"=w405:u8, "Started"=w400:bool)  [unwired: 7 in, 1 out]
        n253 = Array Subset(array=w406, length (row)=w405) -> (w404:string[][])  [unwired: 3 in]
        n254 = Select(t="Executing" ("Cmd Status"), s=w400, f="" ("Cmd Status")) -> (s? t:f=w401:string)
        n255 = local write "Cmd Status"(w401) -> ()
      }
      event "CheckList": Double Click {
        # "Shift clears all"
        # "Update symbols on the listbox"
        n256 = event-data() -> ("PlatMods.Shift"=w414:bool, "Row"=w416:i32)  [unwired: 1 in]
        n257 = case shown="True" w414 {
          tunnel: w416 -> [w420 _]
          tunnel: 1 -> [w419 _]
          frame False {
            n258 = property on="CheckList" class="LstBox (strict)"() -> ("Item Symbols"=w418:i32[])  [unwired: 2 in, 2 out]
            n259 = Replace Array Subset(array=w418, new element=w419, index=w420) -> (w417:i32[])
            n260 = property on="CheckList" class="LstBox (strict)"("Item Symbols"=w417) -> ()  [unwired: 2 in, 2 out]
          }
          frame True {
            w421 = 0 ("Top Row")
            n261 = property on="CheckList" class="LstBox (strict)"() -> ("Number of Rows"=w423:u32)  [unwired: 2 in, 2 out]
            n262 = Initialize Array(0, w423) -> (w422:i32[])
            n263 = property on="CheckList" class="LstBox (strict)"("Top Row"=w421, "Value"=w421, "Item Symbols"=w422) -> ()  [unwired: 2 in, 2 out]
          }
        }
      }
      event "CheckList": Key Down {
        # "Update symbols on the listbox\nLeft and right keys check and uncheck"
        n264 = event-data() -> ("VKey"=w428:T23)  [unwired: 1 in]
        n265 = case shown="\"Left\", \"Right\"" w428 {
          selector: w428 -> [w433 _]
          tunnel: eventvkey."Left" ("VKey") -> [w431 _]
          frame "Left", "Right" {
            n266 = Equal?(x=w431, y=w433) -> (x = y?=w432:bool)
            n267 = Select(t=0, s=w432, f=1) -> (s? t:f=w434:i32)
            n268 = property on="CheckList" class="LstBox (strict)"() -> ("Item Symbols"=w437:i32[])  [unwired: 2 in, 2 out]
            n269 = Replace Array Subset(array=w437, new element=w434, index="CheckList") -> (w436:i32[])
            n270 = property on="CheckList" class="LstBox (strict)"("Item Symbols"=w436) -> ()  [unwired: 2 in, 2 out]
          }
          frame Default {
          }
        }
      }
      event "DB Camera Config": Value Change {
        # "Show or hide the cluster of controls, store in ini file"
        n271 = event-data() -> ("NewVal"=w442:bool)  [unwired: 1 in]
        n272 = case shown="False" w442 {
          tunnel: w441 -> [w451 _]
          tunnel: [w444 w462] -> w440
          tunnel: w439 -> [w443 w462]
          frame False {
            w458 = "Camera"
            w461 = FALSE ("Visible")
            n273 = local read "Camera Settings"() -> (w450:T3)
            n274 = Index Array(array=w451) -> (element=w454:cluster{string[]})  [unwired: 1 in]
            n275 = Unbundle(w450) -> ("Frame Rate"=w449:i32, "Compression"=w448:i32, "Size"=w452:u16)
            n276 = Unbundle(w454) -> (w453:string[])
            n277 = Index Array(array=w453, index=w452) -> (element=w447:string)
            n278 = call-poly <vilib>:"Write Key.vi"("section"=w458, "value"=w447, "key"="Size", "refnum"=w443) -> ("refnum out"=w460:T14)  [unwired: 2 in, 5 out]
            n279 = call-poly <vilib>:"Write Key.vi"("section"=w458, "value"=w449, "key"="FrameRate", "refnum"=w460) -> ("refnum out"=w459:T14)  [unwired: 1 in, 6 out]
            n280 = property on="Camera Settings" class="Clust (strict)"("Visible"=w461) -> ()  [unwired: 2 in, 2 out]
            n281 = local write "DB Camera Config"(w461) -> ()
            n282 = call-poly <vilib>:"Write Key.vi"("section"=w458, "value"=w448, "key"="Compression", "refnum"=w459) -> ("refnum out"=w445:T14)  [unwired: 1 in, 6 out]
            n283 = call <vilib>:"Close Config Data.vi"("refnum"=w445) -> ("file path"=w446:path)  [unwired: 2 in, 8 out]
            n284 = call <vilib>:"Open Config Data.vi"("configuration file path"=w446) -> ("refnum"=w444:T14)  [unwired: 8 in, 2 out]
          }
          frame True {
            n285 = property on="Camera Settings" class="Clust (strict)"("Visible"=TRUE) -> ()  [unwired: 2 in, 2 out]
          }
        }
      }
      event "Camera Settings": Value Change {
        # "Update summary string when any elements of DB camera change"
        n286 = event-data() -> ("NewVal"=w476:T3)  [unwired: 1 in]
        n287 = Index Array(array=w472) -> (element=w471:cluster{string[]})  [unwired: 1 in]
        n288 = Unbundle(w476) -> ("Frame Rate"=w467:i32, "Compression"=w466:i32, "Size"=w469:u16)
        n289 = Unbundle(w471) -> (w470:string[])
        n290 = Index Array(array=w470, index=w469) -> (element=w468:string)
        n291 = Format Into String(format string="%s   %dfps   %d%%", w468, w467, w466) -> (resulting string=w473:string)  [unwired: 2 in, 1 out]
        n292 = Build Array(w473) -> (w474:string[])
        n293 = property on="DB Camera Config" class="Bool (strict)"("Strings [4]"=w474) -> ()  [unwired: 2 in, 2 out]
      }
      event "Motor.Enable": Value Change {
        # "When the test mode otor enable helper is set, update that\ntree row item's value"
        n294 = event-data() -> ("NewVal"=w483:bool)  [unwired: 1 in]
        n295 = Unbundle("Motor") -> ("Value"=w482:dbl)  [unwired: 1 out]
        n296 = Select(t=w482, s=w483, f=0.0) -> (s? t:f=w480:dbl)
        n297 = call <vilib>:"NT Write Number.vi"("Numeric"=w480, "Name"=w479) -> ()  [unwired: 9 in, 1 out]
      }
      event "Test Slider": Value Change {
        # "When the test mode slider helper is set, update that\ntree row item's value"
        n298 = event-data() -> ("NewVal"=w487:dbl)  [unwired: 1 in]
        n299 = call <vilib>:"NT Write Number.vi"("Numeric"=w487, "Name"=w488) -> ()  [unwired: 9 in, 1 out]
      }
      event "On/Off": Value Change {
        # "When the test mode on/off helper value is set, update that\ntree row item's value"
        n300 = event-data() -> ("NewVal"=w493:bool)  [unwired: 1 in]
        n301 = Boolean To (0,1)(Boolean=w493) -> (0, 1=w492:i16)
        n302 = call <vilib>:"NT Write Number.vi"("Numeric"=w492, "Name"=w491) -> ()  [unwired: 9 in, 1 out]
      }
      event "Rev/Fwd": Value Change {
        # "When the test mode helper value for relays is set, update that\ntree row item's value"
        n303 = event-data() -> ("NewVal.Forward"=w502:bool, "NewVal.Reverse"=w501:bool)  [unwired: 1 in]
        n304 = Boolean To (0,1)(Boolean=w502) -> (0, 1=w498:i16)
        n305 = Boolean To (0,1)(Boolean=w501) -> (0, 1=w500:i16)
        n306 = Negate(x=w500) -> (-x=w499:i16)
        n307 = Add(x=w498, y=w499) -> (x+y=w497:i16)
        n308 = call <vilib>:"NT Write Number.vi"("Numeric"=w497, "Name"=w496) -> ()  [unwired: 9 in, 1 out]
      }
      event "Test Ring": Value Change {
        # "When a test mode helper value is selected from the ring,\nset the tree item's variable to the string value"
        n309 = event-data() -> ("NewVal"=w507:u16)  [unwired: 1 in]
        n310 = property on="Test Ring" class="Ring (strict)"() -> ("Strings []"=w508:string[])  [unwired: 2 in, 2 out]
        n311 = Index Array(array=w508, index=w507) -> (element=w506:string)
        n312 = call <vilib>:"NT Write String.vi"("String"=w506, "Name"=w505) -> ()  [unwired: 9 in, 1 out]
      }
      event "Rec Mode": Value Change {
        # "Update globals for recording mode and path to read log from.\nClear when logging and let NetworkTables set path for vision to\nuse."
        n313 = event-data() -> ("NewVal"=w520:enum32{"Stop", "Record", "Playback"})  [unwired: 1 in]
        n314 = global write "WPI_DashboardLogging Global.vi" "Logging Filename"(path "") -> ()
        n315 = global write "WPI_DashboardLogging Global.vi" "Recording"(w520) -> ()
        n316 = case shown="\"Playback\"" w520 {
          tunnel: w519 -> [_ w522 w531]
          tunnel: [_ _ w530] -> w516
          tunnel: [_ _ w529] -> _
          tunnel: w514 -> [_ _ w527]
          tunnel: cluster{i32, i32} {-250, 170} -> [_ _ w526]
          tunnel: [_ _ T24 {"Image Size"=TRUE, "Image Type"=TRUE, "Pixel Value"=TRUE, "ROI Information"=TRUE, "Zoom Factor"=FALSE} ("Image Information Shown:All Elements")] -> w512
          tunnel: [_ _ TRUE ("Zoom Factor")] -> w511
          tunnel: w510 -> [_ _ w523]
          frame Default {
          }
          frame "Stop", "Record" {
            # "Place Window too"
            n317 = invoke class="VI" method="FP.Close"(reference=w522) -> (reference out=w521:refnum<vi>)  [unwired: 2 in, 2 out]
            n318 = invoke class="VI" method="Abort VI"(reference=w521) -> ()  [unwired: 2 in, 3 out]
          }
          frame "Playback" {
            n319 = call "Open Playback Panel.vi"("Offset"=w526, "DB VI Ref"=w527, "Playback in"=w531) -> ("Playback out"=w528:refnum<vi>)  [unwired: 8 in]
            n320 = register-events(w528, w523) -> (reference out=w530:refnum<event-registration>, error out=w529:errorcluster)  [unwired: 2 in]
          }
        }
        n321 = property on="Camera Image" class="ImageControl"("Image Information Shown"=w512, "Image Information Visible"=w511) -> ()  [unwired: 2 in, 2 out]
        n322 = call <vilib>:"WPI_DashboardNT Log FieldName Cache.vi"("Operation"=enum16{"Lookup/Add", "Index", "Clear"}."Clear") -> ()  [unwired: 8 in, 3 out]
      }
      event Panel Close {
        w533 = enum32{"Stop", "Record", "Playback"}."Stop" ("Rec Mode")
        # "Playback window has been closed, abort"
        n323 = event-data() -> ()  [unwired: 1 in, 4 out]
        n324 = local write "Rec Mode"(w533) -> ()
        n325 = global write "WPI_DashboardLogging Global.vi" "Recording"(w533) -> ()
      }
      event Panel Close {
        # "Abort playback window and ourself"
        n326 = event-data() -> ()  [unwired: 1 in, 4 out]
        n327 = invoke class="VI" method="FP.Close"(reference=w539) -> (reference out=w538:refnum<vi>)  [unwired: 2 in, 2 out]
        n328 = invoke class="VI" method="Abort VI"(reference=w538) -> (error out=w537:errorcluster)  [unwired: 2 in, 2 out]
        n329 = invoke class="VI" method="Abort VI"(error in=w537) -> ()  [unwired: 2 in, 3 out]
      }
      event User Event {
        n330 = event-data() -> ("IDs"=w547:cluster{"RPC field ID":u16, "Unique ID":u16}, "String"=w546:string)  [unwired: 1 in]
        n331 = Bundle("IDs"=w547, "String"=w546) -> (w545:T11)  [unwired: 1 in]
        n332 = call <vilib>:"Retrieve RPC Response.vi"("RPC Response"=w545) -> ("Output"=w542:string[][])  [unwired: 10 in]
        n333 = Build Array (concatenate)(w540, w542) -> (w541:string[][])
        n334 = local write "Command Params"(w541) -> ()
        n335 = local write "Cmd Status"("" ("Cmd Status")) -> ()
      }
      event "Vision": Value Change {
        # "Enable/Disable Compression slider.\nHW USB is hard-coded into the camera"
        n336 = event-data() -> ("NewVal"=w554:u16)  [unwired: 1 in]
        n337 = Equal?(x=w554, y=u32 2 ("milliseconds to wait")) -> (x = y?=w552:bool)
        n338 = Select(t=T25."Disabled and Grayed Out" ("Disabled"), s=w552, f=T25."Enabled" ("Disabled")) -> (s? t:f=w549:T25)
        n339 = property on="Compression" class="Slide (strict)"("DisabledEnum"=w549) -> ()  [unwired: 2 in, 2 out]
      }
      event "Tree": Double Click {
        n340 = event-data() -> ("PlatMods"=w559:T28, "Tag"=w558:string)  [unwired: 1 in]
        n341 = Unbundle(w559) -> ("Shift"=w557:bool)  [unwired: 4 out]
        n342 = Not(x=w557) -> (.not. x?=w556:bool)
        n343 = call <vilib>:"NT Update Persistence.vi"("Persistence"=w556, "Name"=w558) -> ()  [unwired: 9 in, 1 out]
      }
    }
  }
  n344 = while {
    tunnel: w50 -> [w563]
    i -> [w566]
    stop <- FALSE stop-if-true
    n345 = Wait (ms)(milliseconds to wait=u32 100) -> ()  [unwired: 1 out]
    n346 = case shown="\"Playback\"" "Rec Mode" {
      tunnel: w566 -> [_ _ w581]
      tunnel: [u32 2829099 ("Base Color") u32 11141120 ("Target Color") w570] -> w562
      frame "Stop", Default {
        # "Reset the color, extra updates don't cost much"
      }
      frame "Record" {
      }
      frame "Playback" {
        # "Playback"
        n347 = Quotient & Remainder(x=w581, y=u32 50 ("milliseconds to wait")) -> (x-y*floor(x/y)=w577:u32)  [unwired: 1 out]
        n348 = Divide(x=w577, y=u32 50 ("milliseconds to wait")) -> (x/y=w574:dbl)
        n349 = Multiply(x=6.283185307179586, y=w574) -> (x*y=w579:dbl)
        n350 = Sine(x=w579) -> (sin(x)=w578:dbl)
        n351 = Absolute Value(x=w578) -> (abs(x)=w571:dbl)
        n352 = call "Interpolate RGB Color.vi"("Proportion"=w571, "Target Color"=u32 30976, "Base Color"=u32 2829099) -> ("Result Color"=w570:u32)  [unwired: 8 in]
      }
    }
    n353 = property class="Pane"(reference=w563, "PaneColor"=w562) -> ()  [unwired: 1 in, 2 out]
  }
  n354 = local write "Dashboard Tab"(T2."Drive" ("Dashboard Tab")) -> ()
  n355 = property on="On/Off" class="Bool (strict)"("Visible"=w18) -> ()  [unwired: 2 in, 2 out]
  n356 = property on="Motor" class="Clust (strict)"("Visible"=w18) -> ()  [unwired: 2 in, 2 out]
  n357 = property on="Progress" class="Clust (strict)"("Visible"=w18) -> ()  [unwired: 2 in, 2 out]
  n358 = property on="Test Ring" class="Ring (strict)"("Visible"=w18) -> ()  [unwired: 2 in, 2 out]
  n359 = property on="Rev/Fwd" class="Clust (strict)"("Visible"=w18) -> ()  [unwired: 2 in, 2 out]
  n360 = property on="Camera Settings" class="Clust (strict)"("Visible"=w18) -> ()  [unwired: 2 in, 2 out]
  n361 = while {
    tunnel: u16 1741 ("timeout ms (25000)") -> [w583]
    stop <- FALSE stop-if-true
    n362 = TCP Create Listener(10:w583) -> (0:w582:errorcluster, 3:w584:refnum<k5>)  [unwired: 4 in, 1 out]
    n363 = case shown="No Error" w582 {
      selector: w582 -> [w586 _]
      tunnel: w584 -> [w587 _]
      frame No Error {
        n364 = while {
          tunnel: w587 -> [w590]
          tunnel: w586 -> [w589]
          stop <- FALSE stop-if-true
          n365 = TCP Wait On Listener(8:w589, 11:w590) -> (0:w591:errorcluster, 4:w592:refnum<k5>)  [unwired: 2 in, 3 out]
          n366 = local write "TCP"(w592) -> ()
          n367 = case shown="No Error" w591 {
            frame No Error {
            }
            frame Error {
              n368 = Wait (ms)(milliseconds to wait=u32 1000) -> ()  [unwired: 1 out]
            }
          }
        }
      }
      frame Error {
        n369 = Wait (ms)(milliseconds to wait=u32 1000) -> ()  [unwired: 1 out]
      }
    }
  }
  n370 = local write "DB Camera Config"(w18) -> ()
  n371 = local write "Command Params"(string[][] [] ("Command Params")) -> ()
  n372 = global write "WPI_DashboardLogging Global.vi" "Recording"(w44) -> ()
  n373 = local write "Command Selection"(u16 0 ("milliseconds to wait")) -> ()
  n374 = local write "Rec Mode"(w44) -> ()
